vi "PS-RA02B FPGA.vi"() -> ()   [LabVIEW 2011]
uses:
  <vilib>/rvi/eio/common/nirviEmuTemplateMethod_errors.vi
  <vilib>/eio/EIONode/EIONode.xnode
  <vilib>/eio/EIOMethodNode/EIOMethodNode.xnode
  Filter VIs.lvlib
panel:
  out "Timestamp":u32 caption="Tick Count(Ticks)"
  out "Mod5/AI0":fxp<+/-,20,5> format="%.17g"
  out "Mod5/AI2":fxp<+/-,20,5> format="%.17g"
  out "Mod5/AI3":fxp<+/-,20,5> format="%.17g"
  out "Mod1/AI0":fxp<+/-,20,5> format="%.17g"
  out "Mod1/AI1":fxp<+/-,20,5> format="%.17g"
  out "Mod1/AI2":fxp<+/-,20,5> format="%.17g"
  out "Mod1/AI3":fxp<+/-,20,5> format="%.17g"
  out "Mod5/AI1":fxp<+/-,20,5> format="%.17g"
  out "period":u32
  out "delay":u32
  out "dperiod":u32
  out "ACH04-Setpoint":fxp<+/-,20,5>
  out "ALV04B-Setpoint":fxp<+/-,20,5>
  out "ACH03B-Setpoint":fxp<+/-,20,5>
  out "ALV04A-Setpoint":fxp<+/-,20,5>
  out "ACV05A-Setpoint":fxp<+/-,20,5>
  out "ACH05A-Setpoint":fxp<+/-,20,5>
  out "ACV03B-Setpoint":fxp<+/-,20,5>
  out "RRA02B-Setpoint":fxp<+/-,20,5>
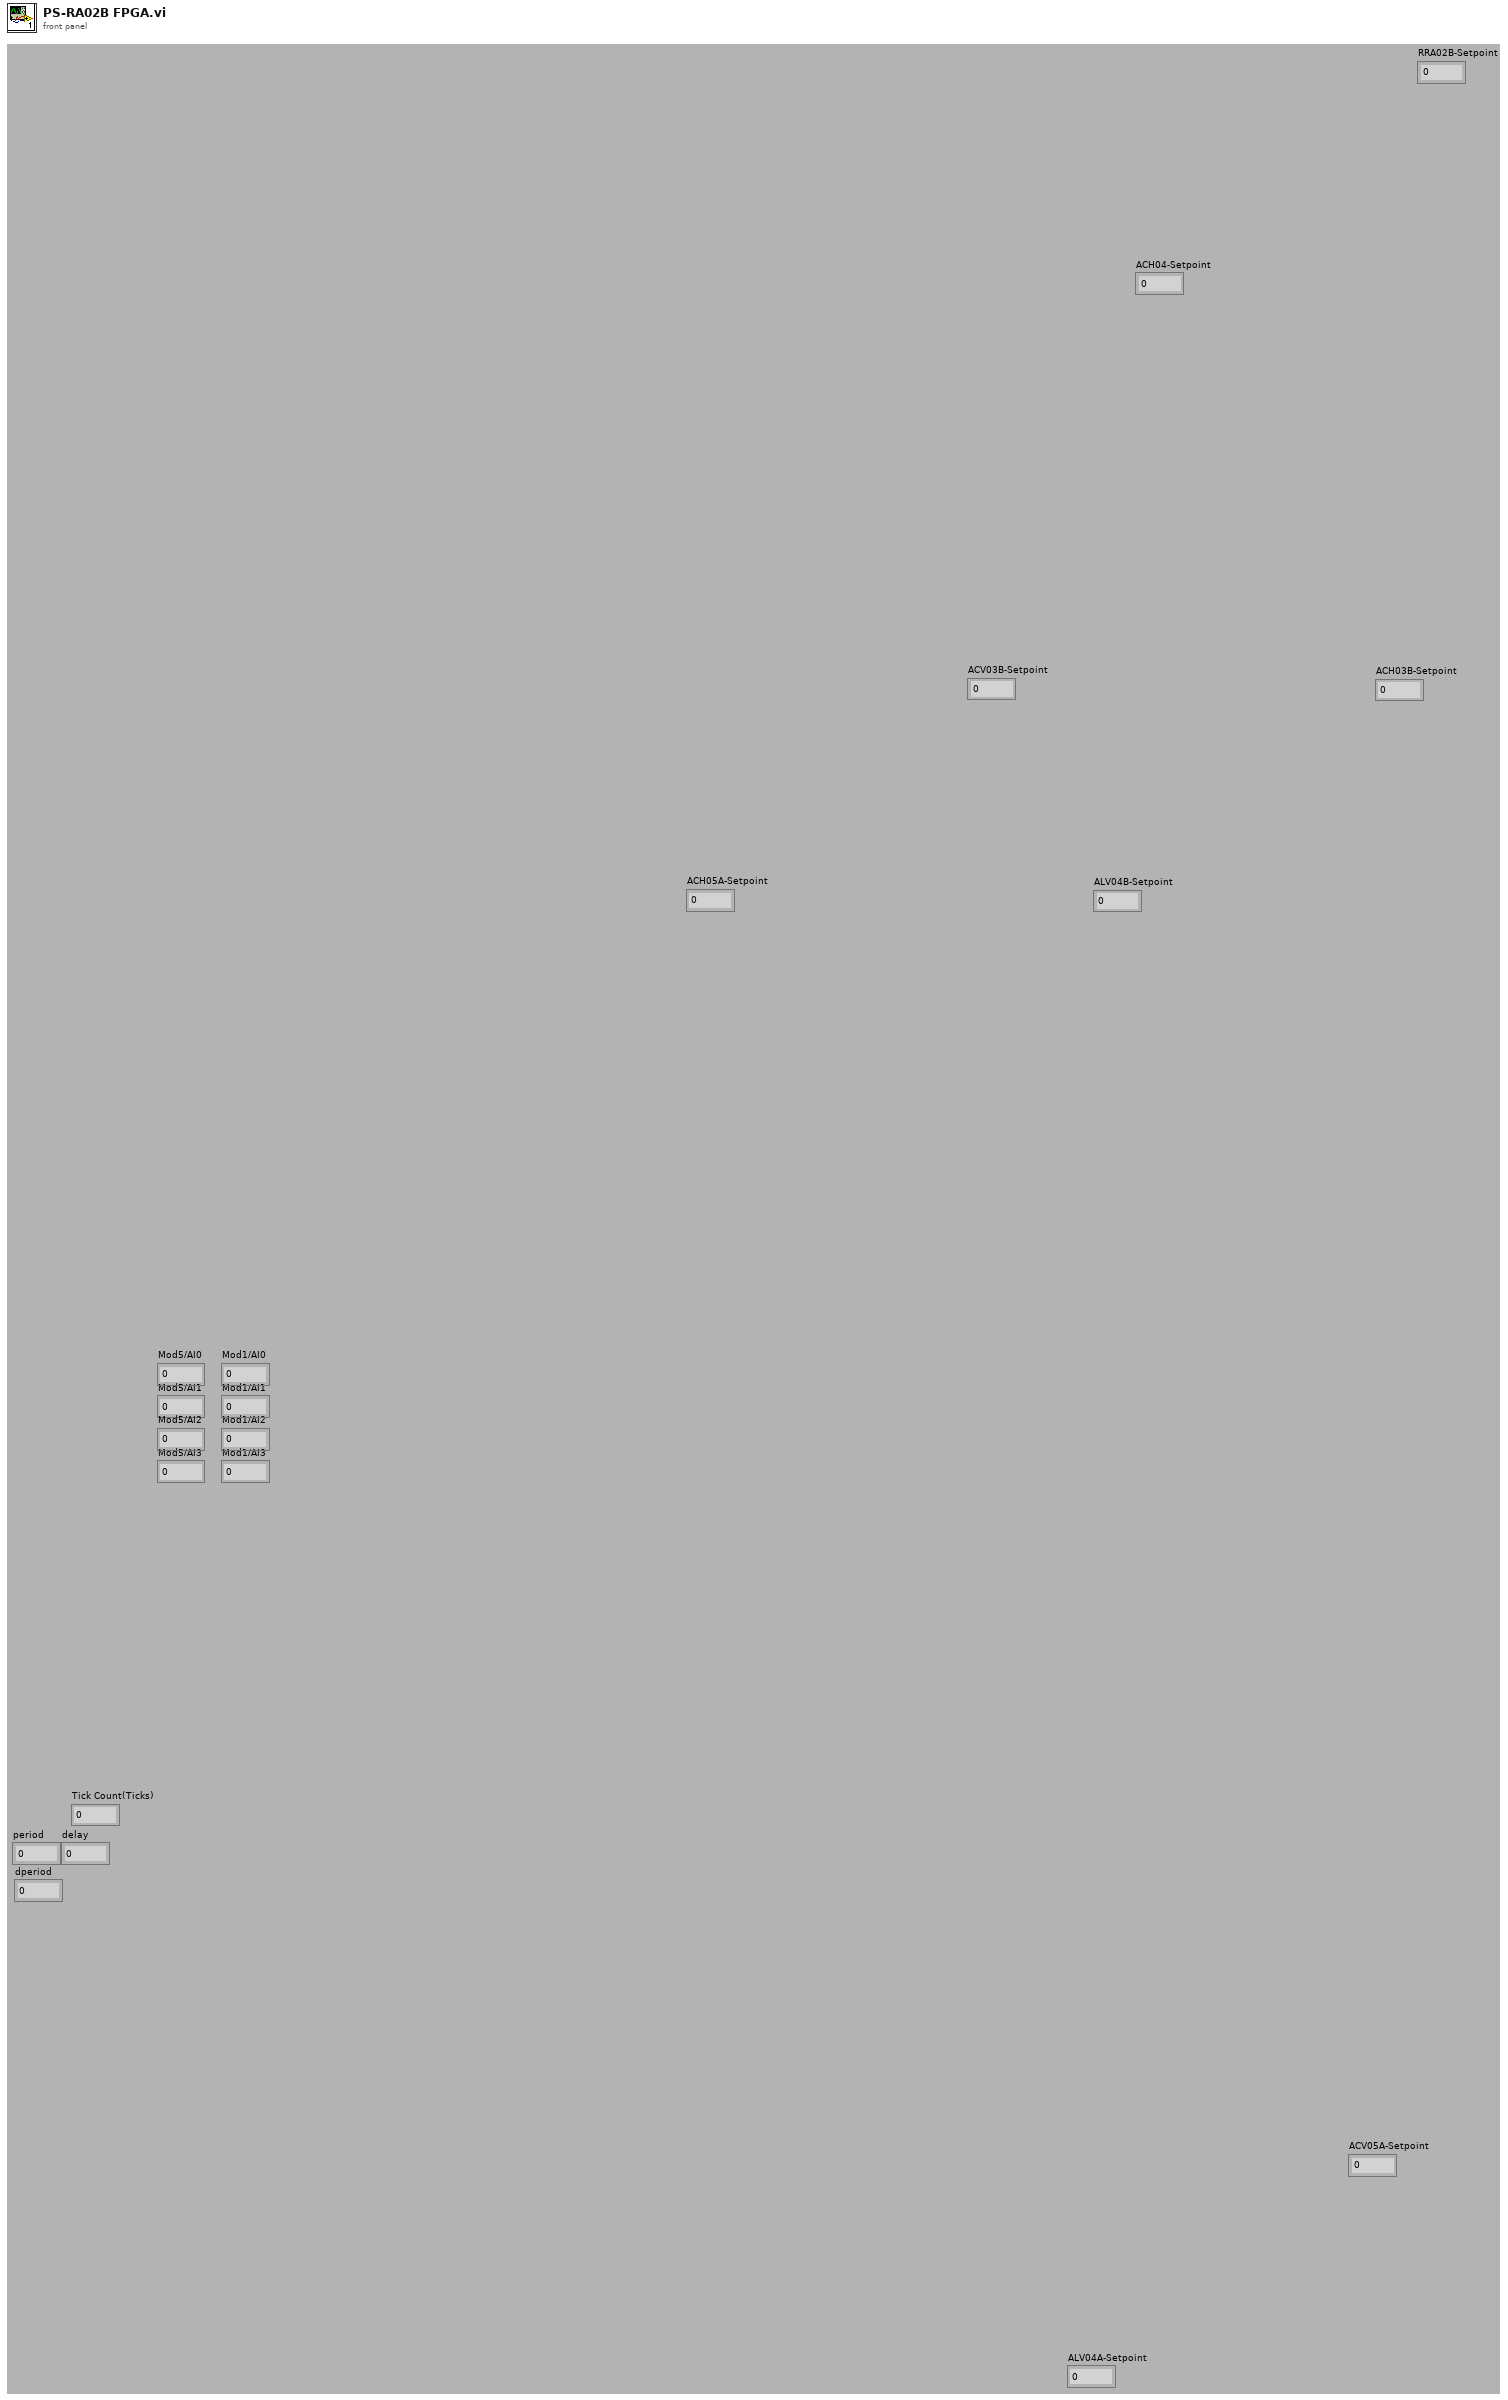
[diagram p1: front panel]
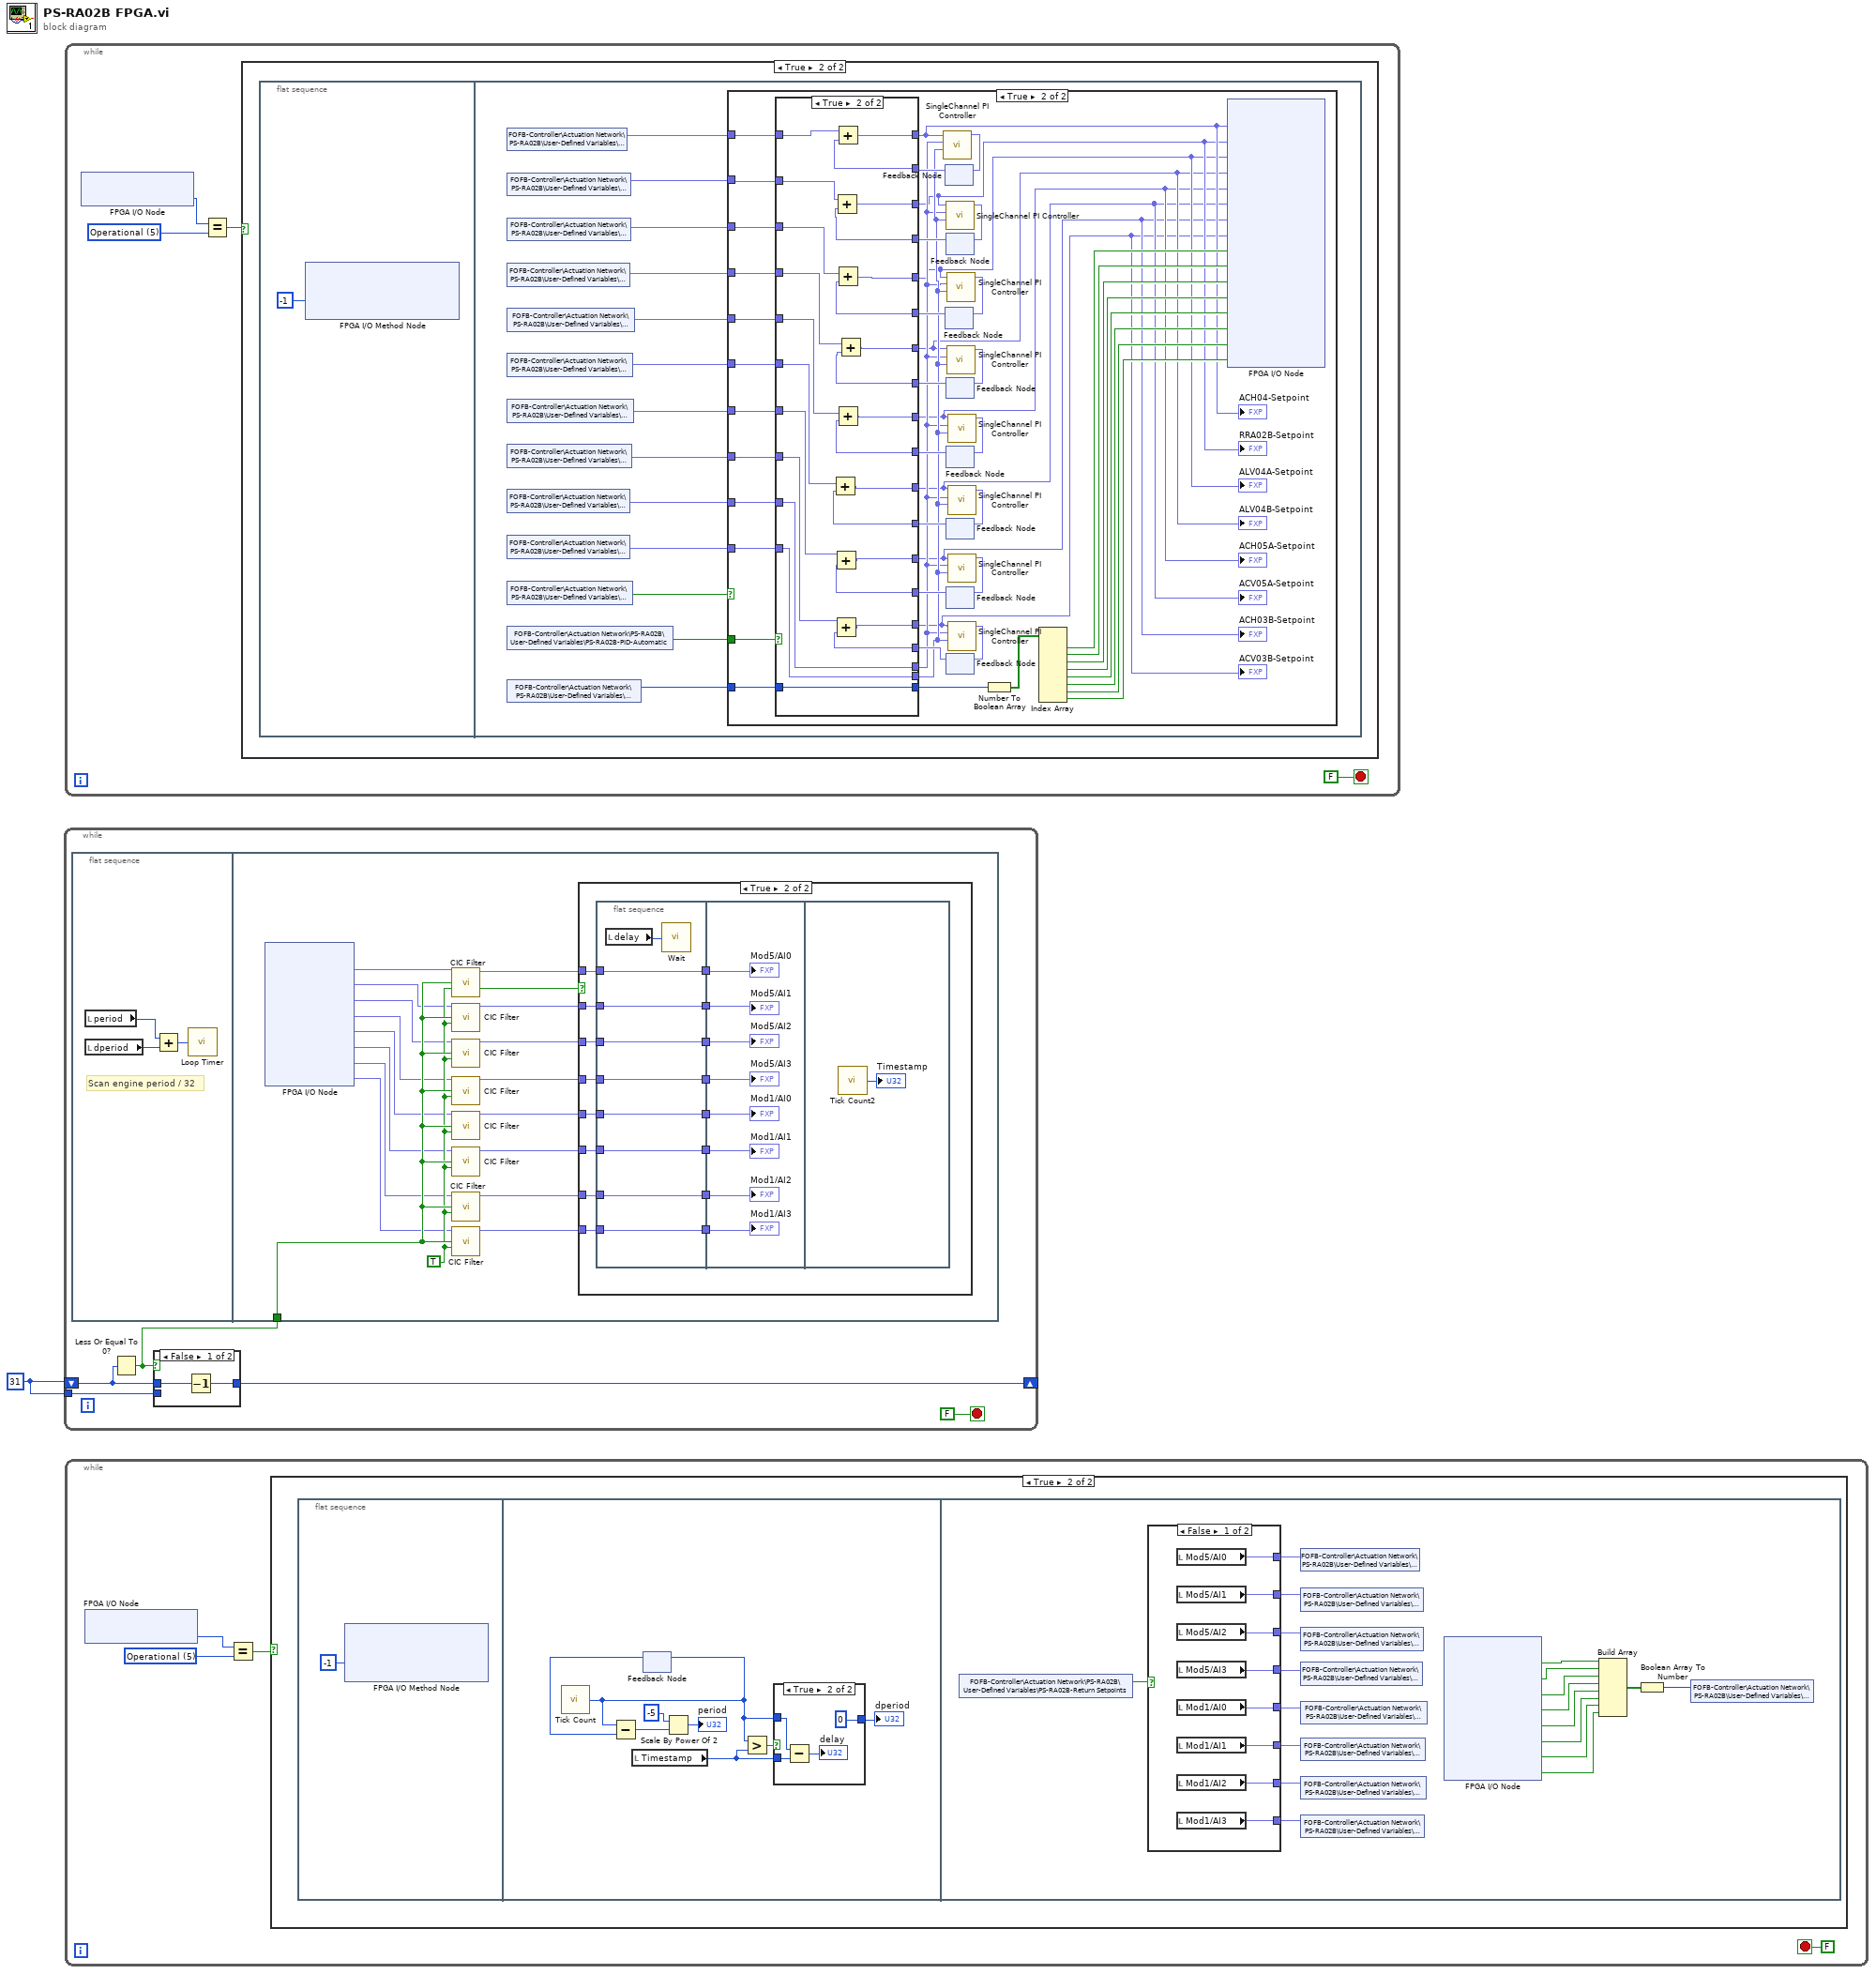
[diagram p0: block diagram]
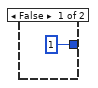
[diagram p5: hidden frame]
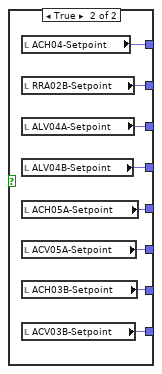
[diagram p6: hidden frame]
diagram:
  w1 = 31
  n1 = while {
    shift-right: [w5] -> _
    shift-left: w1 -> [w4]
    tunnel: w1 -> [w2]
    stop <- FALSE stop-if-true
    n2 = flat-sequence {
      tunnel: w3 -> [w31]
      frame #0 {
        # "Scan engine period / 32"
        n3 = local read "period"() -> (w12:u32)
        n4 = local read "dperiod"() -> (w11:u32)
        n5 = Add(x=w12, y=w11) -> (x+y=w10:u32)
        n6 = call "Loop Timer"("Count(Ticks)"=w10) -> ()  [unwired: 1 out]
      }
      frame #1 {
        w30 = TRUE ("input valid")
        n7 = xnode "FPGA I/O Node"() -> ("Mod5/AI0"=w20:fxp<+/-,20,5>, "Mod5/AI1"=w19:fxp<+/-,20,5>, "Mod5/AI2"=w18:fxp<+/-,20,5>, "Mod5/AI3"=w17:fxp<+/-,20,5>, "Mod1/AI0"=w16:fxp<+/-,20,5>, "Mod1/AI1"=w15:fxp<+/-,20,5>, "Mod1/AI2"=w14:fxp<+/-,20,5>, "Mod1/AI3"=w13:fxp<+/-,20,5>)  [unwired: 8 in, 8 out]
        n8 = call "CIC Filter.vi"("input data"=w20, "sample"=w31, "input valid"=w30) -> ("output data"=w28:fxp<+/-,20,5>, "output valid"=w29:bool)  [unwired: 10 in, 1 out]
        n9 = call "CIC Filter.vi"("input data"=w19, "sample"=w31, "input valid"=w30) -> ("output data"=w27:fxp<+/-,20,5>)  [unwired: 10 in, 2 out]
        n10 = call "CIC Filter.vi"("input data"=w18, "sample"=w31, "input valid"=w30) -> ("output data"=w26:fxp<+/-,20,5>)  [unwired: 10 in, 2 out]
        n11 = call "CIC Filter.vi"("input data"=w17, "sample"=w31, "input valid"=w30) -> ("output data"=w25:fxp<+/-,20,5>)  [unwired: 10 in, 2 out]
        n12 = call "CIC Filter.vi"("input data"=w16, "sample"=w31, "input valid"=w30) -> ("output data"=w24:fxp<+/-,20,5>)  [unwired: 10 in, 2 out]
        n13 = call "CIC Filter.vi"("input data"=w15, "sample"=w31, "input valid"=w30) -> ("output data"=w23:fxp<+/-,20,5>)  [unwired: 10 in, 2 out]
        n14 = call "CIC Filter.vi"("input data"=w14, "sample"=w31, "input valid"=w30) -> ("output data"=w22:fxp<+/-,20,5>)  [unwired: 10 in, 2 out]
        n15 = call "CIC Filter.vi"("input data"=w13, "sample"=w31, "input valid"=w30) -> ("output data"=w21:fxp<+/-,20,5>)  [unwired: 10 in, 2 out]
        n16 = case shown="True" w29 {
          tunnel: w28 -> [_ w47]
          tunnel: w27 -> [_ w45]
          tunnel: w26 -> [_ w43]
          tunnel: w25 -> [_ w42]
          tunnel: w24 -> [_ w39]
          tunnel: w23 -> [_ w37]
          tunnel: w22 -> [_ w35]
          tunnel: w21 -> [_ w33]
          frame False {
          }
          frame True {
            n17 = flat-sequence {
              tunnel: w47 -> [w56]
              tunnel: [w56] -> w46
              tunnel: w45 -> [w54]
              tunnel: [w54] -> w44
              tunnel: w43 -> [w52]
              tunnel: w42 -> [w53]
              tunnel: [w53] -> w41
              tunnel: [w52] -> w40
              tunnel: w39 -> [w51]
              tunnel: [w51] -> w38
              tunnel: w37 -> [w50]
              tunnel: [w50] -> w36
              tunnel: w35 -> [w49]
              tunnel: [w49] -> w34
              tunnel: w33 -> [w48]
              tunnel: [w48] -> w32
              tunnel: w46 -> [w63]
              tunnel: w44 -> [w64]
              tunnel: w41 -> [w62]
              tunnel: w40 -> [w61]
              tunnel: w38 -> [w60]
              tunnel: w36 -> [w59]
              tunnel: w34 -> [w58]
              tunnel: w32 -> [w57]
              frame #0 {
                n18 = local read "delay"() -> (w55:u32)
                n19 = call "Wait"("Count(Ticks)"=w55) -> ()  [unwired: 1 out]
              }
              frame #1 {
                "Mod5/AI0" <- w63
                "Mod5/AI2" <- w61
                "Mod5/AI3" <- w62
                "Mod1/AI0" <- w60
                "Mod1/AI1" <- w59
                "Mod1/AI2" <- w58
                "Mod1/AI3" <- w57
                "Mod5/AI1" <- w64
              }
              frame #2 {
                n20 = call "Tick Count2"() -> ("Tick Count(Ticks)"=→"Timestamp":u32)
              }
            }
          }
        }
      }
    }
    n21 = Less Or Equal To 0?(x=w4) -> (x <= 0?=w3:bool)
    n22 = case shown="False" w3 {
      tunnel: [w8 w9] -> w5
      tunnel: w4 -> [w7 _]
      tunnel: w2 -> [_ w9]
      frame False {
        n23 = Decrement(x=w7) -> (x-1=w8:i32)
      }
      frame True {
      }
    }
  }
  n24 = while {
    stop <- FALSE stop-if-true
    w68 = u8 5 items=["Init"=1, "PreOp"=2, "Bootstrap"=3, "SafeOp"=4, "Operational"=5]
    n25 = xnode "FPGA I/O Node"() -> ("EtherCAT State"=w67:u8)  [unwired: 1 in, 1 out]
    n26 = Equal?(x=w67, y=w68) -> (x = y?=w66:bool)
    n27 = case shown="True" w66 {
      frame False {
      }
      frame True {
        n28 = flat-sequence {
          frame #0 {
            n29 = xnode "FPGA I/O Method Node"("Timeout"=-1) -> ()  [unwired: 1 in, 2 out]
          }
          frame #1 {
            n30 = shared-variable "FOFB-Controller\\Actuation Network\\PS-RA02B\\User-Defined Variables\\ACH04-Setpoint"() -> (w83:fxp<+/-,20,5>)  [unwired: 1 in, 1 out]
            n31 = shared-variable "FOFB-Controller\\Actuation Network\\PS-RA02B\\User-Defined Variables\\RRA02B-Setpoint"() -> (w82:fxp<+/-,20,5>)  [unwired: 1 in, 1 out]
            n32 = shared-variable "FOFB-Controller\\Actuation Network\\PS-RA02B\\User-Defined Variables\\ALV04A-Setpoint"() -> (w81:fxp<+/-,20,5>)  [unwired: 1 in, 1 out]
            n33 = shared-variable "FOFB-Controller\\Actuation Network\\PS-RA02B\\User-Defined Variables\\ALV04B-Setpoint"() -> (w80:fxp<+/-,20,5>)  [unwired: 1 in, 1 out]
            n34 = shared-variable "FOFB-Controller\\Actuation Network\\PS-RA02B\\User-Defined Variables\\ACH05A-Setpoint"() -> (w79:fxp<+/-,20,5>)  [unwired: 1 in, 1 out]
            n35 = shared-variable "FOFB-Controller\\Actuation Network\\PS-RA02B\\User-Defined Variables\\ACV05A-Setpoint"() -> (w78:fxp<+/-,20,5>)  [unwired: 1 in, 1 out]
            n36 = shared-variable "FOFB-Controller\\Actuation Network\\PS-RA02B\\User-Defined Variables\\ACH03B-Setpoint"() -> (w77:fxp<+/-,20,5>)  [unwired: 1 in, 1 out]
            n37 = shared-variable "FOFB-Controller\\Actuation Network\\PS-RA02B\\User-Defined Variables\\ACV03B-Setpoint"() -> (w76:fxp<+/-,20,5>)  [unwired: 1 in, 1 out]
            n38 = shared-variable "FOFB-Controller\\Actuation Network\\PS-RA02B\\User-Defined Variables\\PS-RA02B-PID-I1"() -> (w75:fxp<+/-,18,1>)  [unwired: 1 in, 1 out]
            n39 = shared-variable "FOFB-Controller\\Actuation Network\\PS-RA02B\\User-Defined Variables\\PS-RA02B-PID-I2"() -> (w74:fxp<+/-,18,2>)  [unwired: 1 in, 1 out]
            n40 = shared-variable "FOFB-Controller\\Actuation Network\\PS-RA02B\\User-Defined Variables\\PS-RA02B-Enable"() -> (w71:bool)  [unwired: 1 in, 1 out]
            n41 = shared-variable "FOFB-Controller\\Actuation Network\\PS-RA02B\\User-Defined Variables\\PS-RA02B-PID-Automatic"() -> (w73:bool)  [unwired: 1 in, 1 out]
            n42 = shared-variable "FOFB-Controller\\Actuation Network\\PS-RA02B\\User-Defined Variables\\PS-RA02B-ON-OFF"() -> (w72:u8)  [unwired: 1 in, 1 out]
            n43 = case shown="True" w71 {
              tunnel: w83 -> [_ w103]
              tunnel: w82 -> [_ w102]
              tunnel: w81 -> [_ w101]
              tunnel: w80 -> [_ w100]
              tunnel: w79 -> [_ w99]
              tunnel: w78 -> [_ w98]
              tunnel: w77 -> [_ w97]
              tunnel: w76 -> [_ w96]
              tunnel: w75 -> [_ w95]
              tunnel: w74 -> [_ w94]
              tunnel: w73 -> [_ w93]
              tunnel: w72 -> [_ w92]
              frame False {
              }
              frame True {
                n44 = feedback #1() -> (w129:fxp<+/-,20,5>)  [unwired: 1 in]
                n45 = feedback #2() -> (w127:fxp<+/-,20,5>)  [unwired: 1 in]
                n46 = feedback #3() -> (w128:fxp<+/-,20,5>)  [unwired: 1 in]
                n47 = feedback #4() -> (w126:fxp<+/-,20,5>)  [unwired: 1 in]
                n48 = feedback #5() -> (w125:fxp<+/-,20,5>)  [unwired: 1 in]
                n49 = feedback #6() -> (w124:fxp<+/-,20,5>)  [unwired: 1 in]
                n50 = feedback #7() -> (w123:fxp<+/-,20,5>)  [unwired: 1 in]
                n51 = feedback #8() -> (w122:fxp<+/-,20,5>)  [unwired: 1 in]
                n52 = case shown="True" w93 {
                  tunnel: w92 -> [w142 w169]
                  tunnel: [w142 w169] -> w130
                  tunnel: [w141 w166] -> w91
                  tunnel: w94 -> [w132 w168]
                  tunnel: [w132 w168] -> w113
                  tunnel: w95 -> [w133 w167]
                  tunnel: [w133 w167] -> w112
                  tunnel: [w140 w161] -> w90
                  tunnel: [w139 w158] -> w89
                  tunnel: [w138 w155] -> w88
                  tunnel: [w137 w152] -> w87
                  tunnel: [w136 w151] -> w86
                  tunnel: [w135 w146] -> w85
                  tunnel: [w134 w143] -> w84
                  tunnel: w129 -> [_ w165]
                  tunnel: w103 -> [w141 w164]
                  tunnel: w128 -> [_ w162]
                  tunnel: w127 -> [_ w159]
                  tunnel: w126 -> [_ w156]
                  tunnel: w125 -> [_ w153]
                  tunnel: w124 -> [_ w149]
                  tunnel: w123 -> [_ w147]
                  tunnel: w122 -> [_ w144]
                  tunnel: w96 -> [w134 w145]
                  tunnel: w97 -> [w135 w148]
                  tunnel: w98 -> [w136 w150]
                  tunnel: w99 -> [w137 w154]
                  tunnel: w100 -> [w138 w157]
                  tunnel: w101 -> [w139 w160]
                  tunnel: w102 -> [w140 w163]
                  frame False {
                  }
                  frame True {
                    n53 = Add(x=w150, y=w149) -> (x+y=w151:fxp<+/-,20,5>)
                    n54 = Add(x=w148, y=w147) -> (x+y=w146:fxp<+/-,20,5>)
                    n55 = Add(x=w145, y=w144) -> (x+y=w143:fxp<+/-,20,5>)
                    n56 = Add(x=w163, y=w162) -> (x+y=w161:fxp<+/-,20,5>)
                    n57 = Add(x=w164, y=w165) -> (x+y=w166:fxp<+/-,20,5>)
                    n58 = Add(x=w160, y=w159) -> (x+y=w158:fxp<+/-,20,5>)
                    n59 = Add(x=w154, y=w153) -> (x+y=w152:fxp<+/-,20,5>)
                    n60 = Add(x=w157, y=w156) -> (x+y=w155:fxp<+/-,20,5>)
                  }
                }
                "ACH04-Setpoint" <- w91
                "ALV04B-Setpoint" <- w88
                "ACH03B-Setpoint" <- w85
                "ALV04A-Setpoint" <- w89
                "ACV05A-Setpoint" <- w86
                "ACH05A-Setpoint" <- w87
                "ACV03B-Setpoint" <- w84
                "RRA02B-Setpoint" <- w90
                n61 = call "SingleChannel PI Controller.vi"("Integral Coefficient a[k]"=w113, "Integral Coefficient b[k]"=w112, "input data"=w91) -> ("output data"=w121:fxp<+/-,20,5>)  [unwired: 8 in]
                n62 = feedback-in #1(w121) -> ()
                n63 = call "SingleChannel PI Controller.vi"("Integral Coefficient a[k]"=w113, "Integral Coefficient b[k]"=w112, "input data"=w90) -> ("output data"=w120:fxp<+/-,20,5>)  [unwired: 8 in]
                n64 = feedback-in #3(w120) -> ()
                n65 = call "SingleChannel PI Controller.vi"("Integral Coefficient a[k]"=w113, "Integral Coefficient b[k]"=w112, "input data"=w89) -> ("output data"=w119:fxp<+/-,20,5>)  [unwired: 8 in]
                n66 = feedback-in #2(w119) -> ()
                n67 = call "SingleChannel PI Controller.vi"("Integral Coefficient a[k]"=w113, "Integral Coefficient b[k]"=w112, "input data"=w88) -> ("output data"=w118:fxp<+/-,20,5>)  [unwired: 8 in]
                n68 = feedback-in #4(w118) -> ()
                n69 = call "SingleChannel PI Controller.vi"("Integral Coefficient a[k]"=w113, "Integral Coefficient b[k]"=w112, "input data"=w87) -> ("output data"=w117:fxp<+/-,20,5>)  [unwired: 8 in]
                n70 = feedback-in #5(w117) -> ()
                n71 = call "SingleChannel PI Controller.vi"("Integral Coefficient a[k]"=w113, "Integral Coefficient b[k]"=w112, "input data"=w86) -> ("output data"=w116:fxp<+/-,20,5>)  [unwired: 8 in]
                n72 = feedback-in #6(w116) -> ()
                n73 = call "SingleChannel PI Controller.vi"("Integral Coefficient a[k]"=w113, "Integral Coefficient b[k]"=w112, "input data"=w85) -> ("output data"=w115:fxp<+/-,20,5>)  [unwired: 8 in]
                n74 = feedback-in #7(w115) -> ()
                n75 = call "SingleChannel PI Controller.vi"("Integral Coefficient a[k]"=w113, "Integral Coefficient b[k]"=w112, "input data"=w84) -> ("output data"=w114:fxp<+/-,20,5>)  [unwired: 8 in]
                n76 = feedback-in #8(w114) -> ()
                n77 = Number To Boolean Array(number=w130) -> (Boolean array=w131:bool[])
                n78 = Index Array(array=w131) -> (element #1=w111:bool, element #2=w110:bool, element #3=w109:bool, element #4=w108:bool, element #5=w107:bool, element #6=w106:bool, element #7=w105:bool, element #8=w104:bool)  [unwired: 8 in]
                n79 = xnode "FPGA I/O Node"("Mod6/AO0"=w91, "Mod6/AO1"=w90, "Mod6/AO2"=w89, "Mod6/AO3"=w88, "Mod2/AO0"=w87, "Mod2/AO1"=w86, "Mod2/AO2"=w85, "Mod2/AO3"=w84, "Mod4/DIO6"=w111, "Mod4/DIO7"=w110, "Mod4/DIO4"=w109, "Mod4/DIO5"=w108, "Mod4/DIO2"=w107, "Mod4/DIO3"=w106, "Mod4/DIO0"=w105, "Mod4/DIO1"=w104) -> ()  [unwired: 16 in, 16 out]
              }
            }
          }
        }
      }
    }
  }
  n80 = while {
    stop <- FALSE stop-if-true
    w172 = u8 5 items=["Init"=1, "PreOp"=2, "Bootstrap"=3, "SafeOp"=4, "Operational"=5]
    n81 = xnode "FPGA I/O Node"() -> ("EtherCAT State"=w171:u8)  [unwired: 1 in, 1 out]
    n82 = Equal?(x=w171, y=w172) -> (x = y?=w170:bool)
    n83 = case shown="True" w170 {
      frame False {
      }
      frame True {
        n84 = flat-sequence {
          frame #0 {
            n85 = xnode "FPGA I/O Method Node"("Timeout"=-1) -> ()  [unwired: 1 in, 2 out]
          }
          frame #1 {
            n86 = call "Tick Count"() -> ("Tick Count(Ticks)"=w176:u32)
            n87 = local read "Timestamp"() -> (w178:u32)
            n88 = feedback #9() -> (w175:u32)  [unwired: 1 in]
            n89 = Subtract(x=w176, y=w175) -> (x-y=w181:u32)
            n90 = feedback-in #9(w176) -> ()
            n91 = Scale By Power Of 2(n=i8 -5, x=w181) -> (x*2^n=→"period":u32)
            n92 = Greater?(x=w176, y=w178) -> (0:w179:bool)
            n93 = case shown="True" w179 {
              tunnel: w176 -> [_ w187]
              tunnel: w178 -> [_ w186]
              tunnel: [u32 1 ("dt 2") u32 0 ("dt 2")] -> w177
              frame False {
              }
              frame True {
                n94 = Subtract(x=w187, y=w186) -> (x-y=→"delay":u32)
              }
            }
            "dperiod" <- w177
          }
          frame #2 {
            n95 = shared-variable "FOFB-Controller\\Actuation Network\\PS-RA02B\\User-Defined Variables\\PS-RA02B-Return Setpoints"() -> (w197:bool)  [unwired: 1 in, 1 out]
            n96 = case shown="False" w197 {
              tunnel: [w214 w222] -> w195
              tunnel: [w213 w221] -> w194
              tunnel: [w212 w220] -> w193
              tunnel: [w211 w219] -> w192
              tunnel: [w210 w218] -> w191
              tunnel: [w209 w217] -> w190
              tunnel: [w208 w215] -> w189
              tunnel: [w207 w216] -> w188
              frame False {
                n97 = local read "Mod5/AI0"() -> (w214:fxp<+/-,20,5>)
                n98 = local read "Mod5/AI1"() -> (w213:fxp<+/-,20,5>)
                n99 = local read "Mod5/AI2"() -> (w212:fxp<+/-,20,5>)
                n100 = local read "Mod5/AI3"() -> (w211:fxp<+/-,20,5>)
                n101 = local read "Mod1/AI0"() -> (w210:fxp<+/-,20,5>)
                n102 = local read "Mod1/AI1"() -> (w209:fxp<+/-,20,5>)
                n103 = local read "Mod1/AI2"() -> (w208:fxp<+/-,20,5>)
                n104 = local read "Mod1/AI3"() -> (w207:fxp<+/-,20,5>)
              }
              frame True {
                n105 = local read "ACH04-Setpoint"() -> (w222:fxp<+/-,20,5>)
                n106 = local read "RRA02B-Setpoint"() -> (w221:fxp<+/-,20,5>)
                n107 = local read "ALV04A-Setpoint"() -> (w220:fxp<+/-,20,5>)
                n108 = local read "ALV04B-Setpoint"() -> (w219:fxp<+/-,20,5>)
                n109 = local read "ACH05A-Setpoint"() -> (w218:fxp<+/-,20,5>)
                n110 = local read "ACV05A-Setpoint"() -> (w217:fxp<+/-,20,5>)
                n111 = local read "ACH03B-Setpoint"() -> (w215:fxp<+/-,20,5>)
                n112 = local read "ACV03B-Setpoint"() -> (w216:fxp<+/-,20,5>)
              }
            }
            n113 = shared-variable "FOFB-Controller\\Actuation Network\\PS-RA02B\\User-Defined Variables\\ACH04-Reading"(w195) -> ()  [unwired: 1 in, 1 out]
            n114 = shared-variable "FOFB-Controller\\Actuation Network\\PS-RA02B\\User-Defined Variables\\RRA02B-Reading"(w194) -> ()  [unwired: 1 in, 1 out]
            n115 = shared-variable "FOFB-Controller\\Actuation Network\\PS-RA02B\\User-Defined Variables\\ALV04A-Reading"(w193) -> ()  [unwired: 1 in, 1 out]
            n116 = shared-variable "FOFB-Controller\\Actuation Network\\PS-RA02B\\User-Defined Variables\\ALV04B-Reading"(w192) -> ()  [unwired: 1 in, 1 out]
            n117 = shared-variable "FOFB-Controller\\Actuation Network\\PS-RA02B\\User-Defined Variables\\ACH05A-Reading"(w191) -> ()  [unwired: 1 in, 1 out]
            n118 = shared-variable "FOFB-Controller\\Actuation Network\\PS-RA02B\\User-Defined Variables\\ACV05A-Reading"(w190) -> ()  [unwired: 1 in, 1 out]
            n119 = shared-variable "FOFB-Controller\\Actuation Network\\PS-RA02B\\User-Defined Variables\\ACH03B-Reading"(w189) -> ()  [unwired: 1 in, 1 out]
            n120 = shared-variable "FOFB-Controller\\Actuation Network\\PS-RA02B\\User-Defined Variables\\ACV03B-Reading"(w188) -> ()  [unwired: 1 in, 1 out]
            n121 = xnode "FPGA I/O Node"() -> ("Mod3/DIO6"=w205:bool, "Mod3/DIO7"=w204:bool, "Mod3/DIO4"=w203:bool, "Mod3/DIO5"=w202:bool, "Mod3/DIO2"=w201:bool, "Mod3/DIO3"=w200:bool, "Mod3/DIO0"=w199:bool, "Mod3/DIO1"=w198:bool)  [unwired: 8 in, 8 out]
            n122 = Build Array(w205, w204, w203, w202, w201, w200, w199, w198) -> (w206:bool[])
            n123 = Boolean Array To Number(Boolean array=w206) -> (number=w196:u8)
            n124 = shared-variable "FOFB-Controller\\Actuation Network\\PS-RA02B\\User-Defined Variables\\PS-RA02B-Status"(w196) -> ()  [unwired: 1 in, 1 out]
          }
        }
      }
    }
  }
